vi "fpga_W&R_ADCs_W_3DAC_CLK_then_Write.vi"() -> ()   [LabVIEW 2018]
uses:
  <vilib>/rvi/Emulation/niFpgaGetClockAttributes.vi
  <vilib>/rvi/Emulation/niFpgaSctlEmulationGetInTimedLoop.vi
  <vilib>/rvi/Emulation/niFpgaEmulationReportErrorSimple.vi
  <vilib>/rvi/eio/common/nirviEmuTemplateMethod_errors.vi
  <vilib>/rvi/Emulation/niFpgaCriticalErrorInLSC.vi
  <vilib>/eio/EIONode/EIONode.xnode
panel:
  in  "DAC 1 write":bool[](array[boolean])=[FALSE, TRUE, TRUE, TRUE, TRUE, TRUE, TRUE, TRUE, TRUE, TRUE, TRUE, TRUE, TRUE, TRUE, TRUE, TRUE]
  out "ADC read":bool[](array[boolean])=[FALSE, FALSE, FALSE, TRUE, TRUE, TRUE, FALSE, TRUE, FALSE, TRUE, FALSE, FALSE, FALSE, TRUE, FALSE, FALSE]
  in  "ADC write":bool[](array[boolean])=[FALSE, FALSE, FALSE, FALSE, FALSE, TRUE, FALSE, FALSE, FALSE, FALSE, FALSE, FALSE, FALSE, FALSE, FALSE, FALSE]
  in  "delay (us)":u32=40000
  in  "Stop":bool
  in  "DAC 2 write":bool[](array[boolean])=[FALSE, TRUE, TRUE, TRUE, TRUE, TRUE, TRUE, TRUE, TRUE, TRUE, TRUE, TRUE, TRUE, TRUE, TRUE, TRUE]
  in  "DAC 3 write":bool[](array[boolean])=[FALSE, TRUE, TRUE, TRUE, TRUE, TRUE, TRUE, TRUE, TRUE, TRUE, TRUE, TRUE, TRUE, TRUE, TRUE, TRUE]
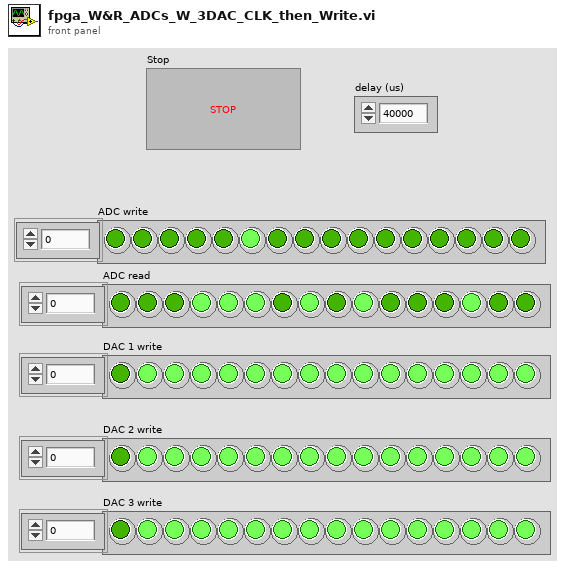
[diagram p1: front panel]
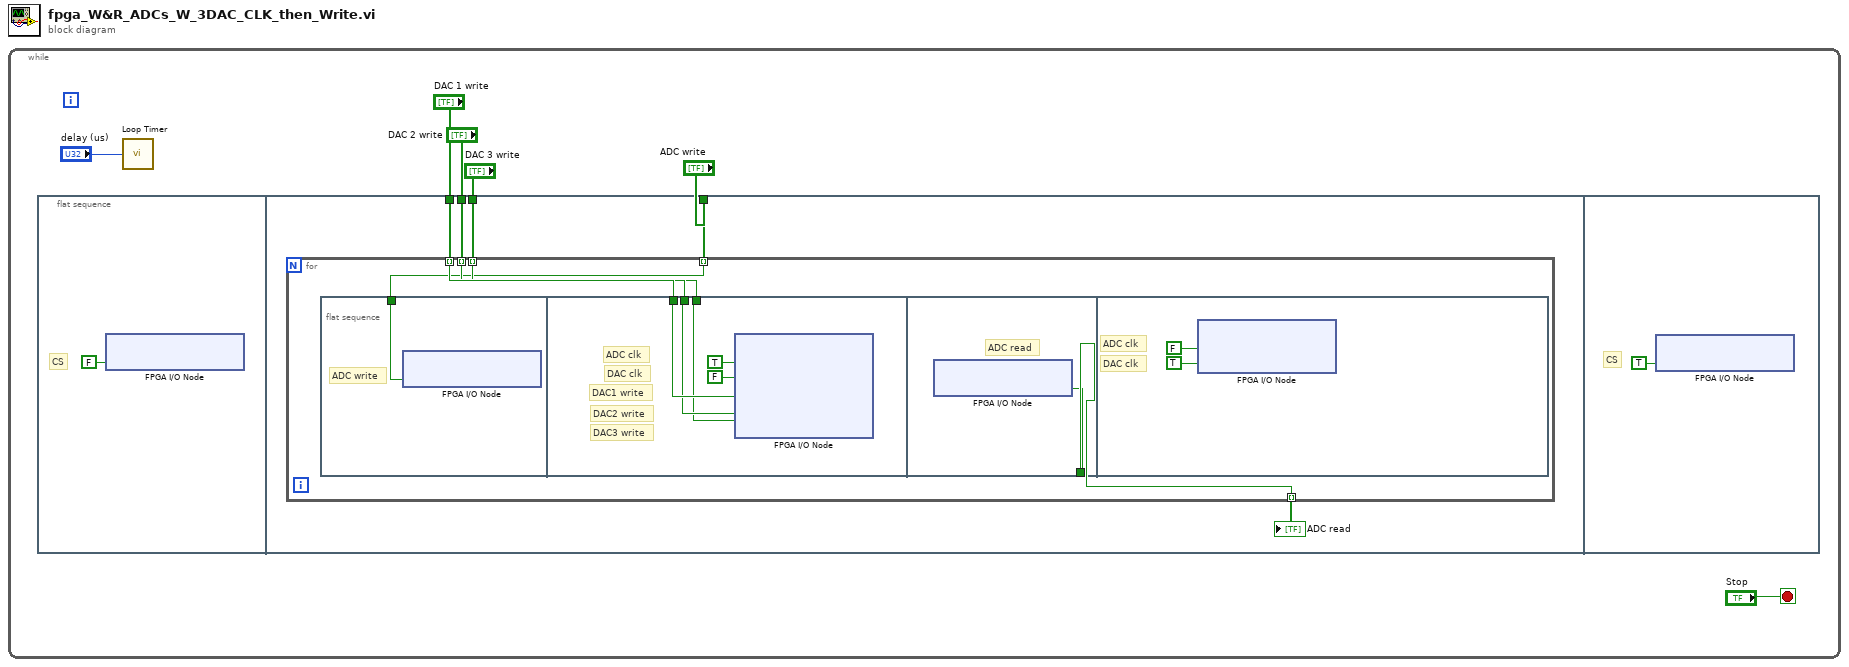
[diagram p0: block diagram]
diagram:
  n1 = while {
    stop <- "Stop" stop-if-true
    n2 = flat-sequence {
      tunnel: "DAC 1 write" -> [w12]
      tunnel: "ADC write" -> [w11]
      tunnel: "DAC 2 write" -> [w9]
      tunnel: "DAC 3 write" -> [w8]
      frame #0 {
        # "CS"
        n3 = xnode "FPGA I/O Node"("ConnectorA/DIO4"=FALSE) -> ()  [unwired: 1 in, 1 out]
      }
      frame #1 {
        n4 = for {
          tunnel: w12 -> [w17] mode=indexing
          tunnel: w11 -> [w14] mode=indexing
          tunnel: [w13] -> w10 mode=indexing
          tunnel: w9 -> [w16] mode=indexing
          tunnel: w8 -> [w15] mode=indexing
          n5 = flat-sequence {
            tunnel: w14 -> [w18]
            tunnel: w17 -> [w21]
            tunnel: w16 -> [w20]
            tunnel: w15 -> [w19]
            tunnel: [w24] -> w13
            frame #0 {
              # "ADC write"
              n6 = xnode "FPGA I/O Node"("ConnectorA/DIO2"=w18) -> ()  [unwired: 1 in, 1 out]
            }
            frame #1 {
              # "DAC3 write"
              # "DAC2 write"
              # "DAC1 write"
              # "DAC clk"
              # "ADC clk"
              n7 = xnode "FPGA I/O Node"("ConnectorA/DIO3"=TRUE, "ConnectorA/DIO5"=FALSE, "ConnectorA/DIO6"=w21, "ConnectorA/DIO7"=w20, "ConnectorA/DIO8"=w19) -> ()  [unwired: 5 in, 5 out]
            }
            frame #2 {
              # "ADC read"
              n8 = xnode "FPGA I/O Node"() -> ("ConnectorA/DIO1"=w24:bool)  [unwired: 1 in, 1 out]
            }
            frame #3 {
              # "DAC clk"
              # "ADC clk"
              n9 = xnode "FPGA I/O Node"("ConnectorA/DIO3"=FALSE, "ConnectorA/DIO5"=TRUE) -> ()  [unwired: 2 in, 2 out]
            }
          }
        }
        "ADC read" <- w10
      }
      frame #2 {
        # "CS"
        n10 = xnode "FPGA I/O Node"("ConnectorA/DIO4"=TRUE) -> ()  [unwired: 1 in, 1 out]
      }
    }
    n11 = call "Loop Timer"("Count(Ticks)"="delay (us)") -> ()  [unwired: 1 out]
  }
